vi "GetName.vi"(5 "base name":string, 7 "add self":bool=TRUE, 8 "error in":errorcluster, 11 "GObj Refnum":refnum<vi>) -> (0 "error out":errorcluster, 2 "UID":string, 3 "name":string)   [LabVIEW 2014, in "Python Functions.lvlib"]
uses:
  Python Functions.lvlib
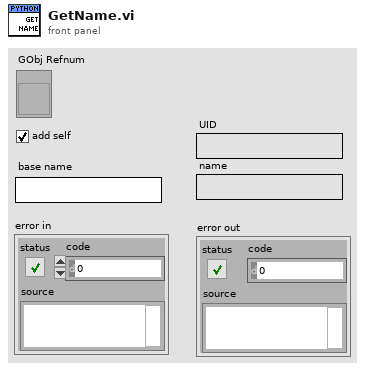
[diagram p1: front panel]
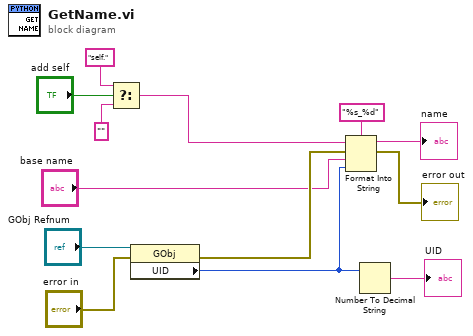
[diagram p0: block diagram]
diagram:
  n1 = Select(t="self." ("format string"), s="add self", f="") -> (s? t:f=w6:string)
  n2 = property class="GObj"(reference="GObj Refnum", error in="error in") -> (error out=w10:errorcluster, "UID"=w3:i32)  [unwired: 1 out]
  n3 = Format Into String(format string="%s_%d", initial string=w6, error in=w10, "base name", w3) -> (resulting string=→"name":string, error out=→"error out":errorcluster)
  n4 = Number To Decimal String(number=w3) -> (decimal integer string=→"UID":string)  [unwired: 1 in]
